vi "二维码识别.vi"() -> ()   [LabVIEW 2018]
uses:
  <vilib>/userdefined/High Color/IMAQdx.ctl
  <vilib>/vision/driver/NI_Vision_Acquisition_Software.lvlib
  <vilib>/vision/NI_Vision_Development_Module.lvlib
panel:
  in  "停止":bool
  out "Data":string
  out "Image":T1(plugin-control)
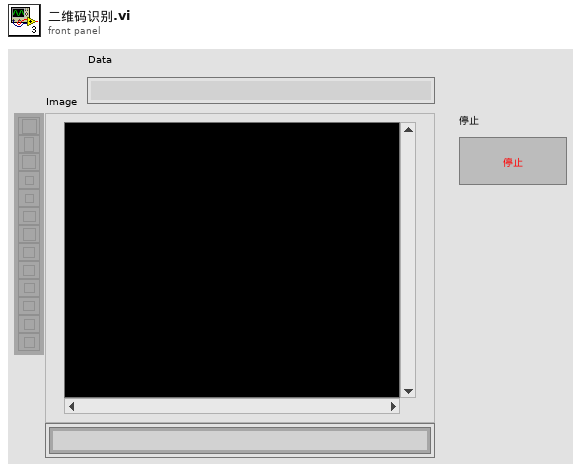
[diagram p1: front panel]
types:
  T1 = typedef "IMAQ Image.ctl" = refnum<image>
  T2 = typedef "IMAQdx.ctl" = refnum<k21>
  T3 = cluster{"Data":string, "Special Char 1":string, "Special Char 2":string, "Checksum(s)":string, "Barcode Type":u32, "Confidence Level":sgl, "Bounding Box":cluster{"x":sgl, "y":sgl}[]}[]
  T4 = cluster{"Data":string, "Special Char 1":string, "Special Char 2":string, "Checksum(s)":string, "Barcode Type":u32, "Confidence Level":sgl, "Bounding Box":cluster{"x":sgl, "y":sgl}[]}
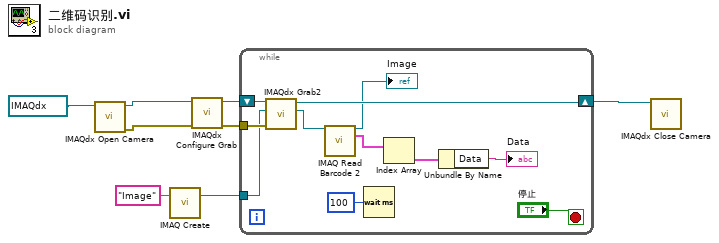
[diagram p0: block diagram]
diagram:
  n1 = call <vilib>:"IMAQdx Open Camera.vi"("Session In"=T2 "cam0") -> ("error out"=w6:errorcluster, "Session Out"=w8:T2)  [unwired: 9 in]
  n2 = call "IMAQ Create"("Image Name"="Image") -> ("New Image"=w2:T1)  [unwired: 4 in, 1 out]
  n3 = call <vilib>:"IMAQdx Configure Grab.vi"("error in"=w6, "Session In"=w8) -> ("error out"=w5:errorcluster, "Session Out"=w7:T2)  [unwired: 8 in]
  n4 = while {
    tunnel: w5 -> [w18]
    shift-right: [w17] -> w4
    shift-left: w7 -> [w19]
    tunnel: w2 -> [w15]
    stop <- "停止" stop-if-true
    n5 = call <vilib>:"IMAQdx Grab2.vi"("error in"=w18, "Image In"=w15, "Session In"=w19) -> ("Image Out"=w14:T1, "Session Out"=w17:T2)  [unwired: 5 in, 2 out]
    n6 = call "IMAQ Read Barcode 2"("Image"=w14) -> ("Image (duplicate)"=→"Image":T1, "Barcodes"=w12:T3)  [unwired: 10 in, 3 out]
    n7 = Wait (ms)(milliseconds to wait=u32 100 ("等待时间（毫秒）")) -> ()  [unwired: 1 out]
    n8 = Index Array(array=w12) -> (element=w11:T4)  [unwired: 1 in]
    n9 = Unbundle By Name(w11) -> ("Data"=→"Data":string)
  }
  n10 = call <vilib>:"IMAQdx Close Camera.vi"("Session In"=w4) -> ()  [unwired: 10 in, 1 out]
